vi "WriteConfig.vi"(8 "error in (no error)":errorcluster, 10 "Config":variant, 11 "PmuCalCal in":refnum<class "PmuCalCal.lvclass">) -> (0 "error out":errorcluster, 3 "PmuCalCal out":refnum<class "PmuCalCal.lvclass">)   [LabVIEW 2018, in "SensorPlugins.lvlib" / "PmuCalCal.lvclass"]
uses:
  PmuCalCal.lvclass
  PmuBaseClass/PmuBase.lvclass
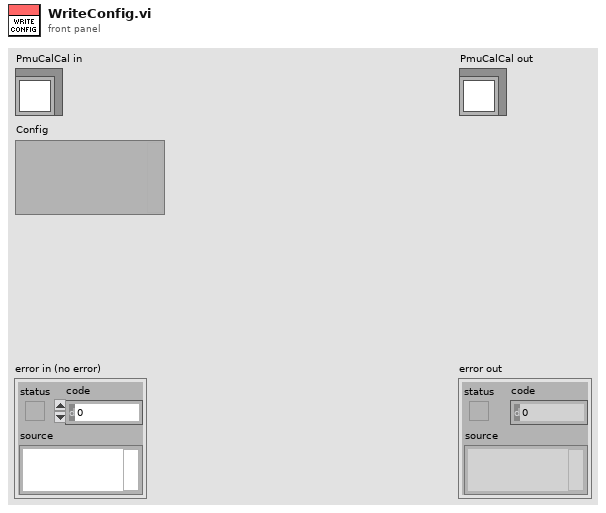
[diagram p1: front panel]
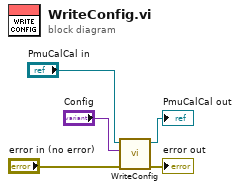
[diagram p0: block diagram]
diagram:
  n1 = call-parent "WriteConfig.vi"("error in (no error)"="error in (no error)", "Config"="Config", "PmuBase in"="PmuCalCal in") -> ("error out"=→"error out":errorcluster, "PmuBase out"=→"PmuCalCal out":refnum<class "PmuCalCal.lvclass">)  [unwired: 7 in]
